vi "HHMI - Filepaths global.vi"() -> ()   [LabVIEW 2013]
doc: "All directory and file paths are stored in this global."
panel:
  in  ".ini path":path
  in  "Simulation filepath":path
  in  "Project dir":path
  # "MAIN"
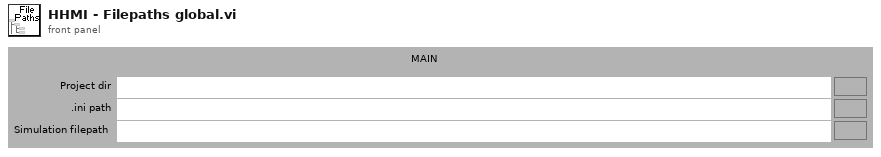
[diagram p1: front panel]
diagram:
